vi "CombineCodes.vi"(9 "BP Main":T1, 10 "Spike Main":T1) -> (2 "Combined":T2)   [LabVIEW 2016]
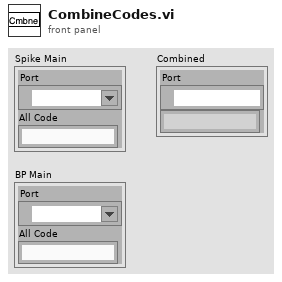
[diagram p1: front panel]
types:
  T1 = cluster{"Port":refnum<visa-resource-name>, "All Code":string}
  T2 = cluster{"Port":refnum<visa-resource-name>, string}
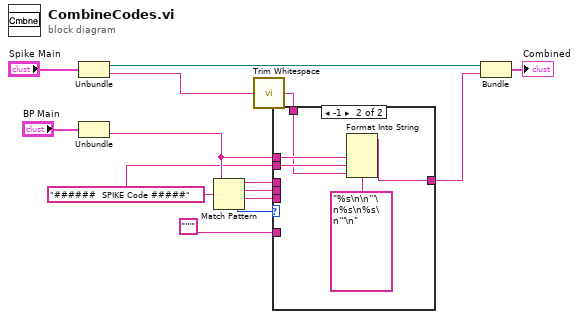
[diagram p0: block diagram]
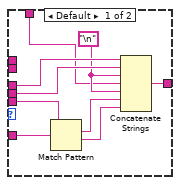
[diagram p2: hidden frame]
diagram:
  w1 = "######  SPIKE Code #####" ("regular expression")
  n1 = Unbundle("Spike Main") -> ("Port"=w13:refnum<visa-resource-name>, "All Code"=w7:string)
  n2 = Unbundle("BP Main") -> ("All Code"=w2:string)  [unwired: 1 out]
  n3 = Match Pattern(string=w2, regular expression=w1) -> (before substring=w8:string, match substring=w6:string, after substring=w10:string, offset past match=w3:i32)  [unwired: 1 in]
  n4 = call <vilib>:"Trim Whitespace.vi"("string"=w7) -> ("trimmed string"=w5:string)  [unwired: 1 in]
  n5 = case shown="-1" w3 {
    tunnel: w10 -> [w23 _]
    tunnel: "'''" ("regular expression") -> [w22 _]
    tunnel: w8 -> [w21 _]
    tunnel: w6 -> [w20 _]
    tunnel: w5 -> [w17 w25]
    tunnel: [w16 w24] -> w4
    tunnel: w2 -> [_ w27]
    tunnel: w1 -> [_ w26]
    frame Default {
      w18 = "\n"
      n6 = Match Pattern(string=w23, regular expression=w22) -> (match substring=w19:string, after substring=w15:string)  [unwired: 1 in, 2 out]
      n7 = Concatenate Strings(w21, w20, w18, w17, w18, w19, w15) -> (w16:string)
    }
    frame -1 {
      n8 = Format Into String(format string="%s\n\n'''\n%s\n%s\n'''\n", w27, w26, w25) -> (resulting string=w24:string)  [unwired: 2 in, 1 out]
    }
  }
  n9 = Bundle("Port"=w13, w4) -> (→"Combined":T2)  [unwired: 1 in]
